vi "Finish.vi"   [LabVIEW 2012]
doc: "This VI is called just before exiting. It is expected to close I/O refnum, save collected data, etc."
uses:
  <vilib>/Rock Robotics/WPI/RobotDrive/WPI_RobotDriveGetSetRefNum.vi
  <vilib>/Rock Robotics/WPI/Joystick/WPI_JoystickGetSetRefNum.vi
types:
  T1 = typedef "WPI_SolenoidDevRef.ctl" = cluster{"DevStatus":errorcluster, "Solenoid Module":T2, "Forward Solenoid Channel":T3, "Reverse Solenoid Channel":T3}
  T2 = typedef "FPGA_TypedefSolenoidModule.ctl" = enum16{"Solenoid Module 1", "Solenoid Module 2"}
  T3 = typedef "WPI_SolenoidChannel.ctl" = enum8{"Solenoid 1", "Solenoid 2", "Solenoid 3", "Solenoid 4", "Solenoid 5", "Solenoid 6", "Solenoid 7", "Solenoid 8", "Invalid"}
  T4 = typedef "WPI_JoystickDevRef.ctl" = cluster{"Device":T5}
  T5 = typedef "WPI_JoystickDeviceEnum.ctl" = enum16{"USB 1", "USB 2", "USB 3", "USB 4", "Kinect 1", "Kinect 2"}
  T6 = typedef "WPI_RobotDriveDevRef.ctl" = cluster{"DevStatus":errorcluster, "Motors[]":T7[], "Square Inputs":bool, "Max Output":dbl, "Isochronous":bool}
  T7 = typedef "WPI_MotorControlDeviceRef.ctl" = cluster{"DeviceStatus":errorcluster, "Type":enum16{"PWM", "CAN"}, "PWM":cluster{"Digital Module":T8, "PWM Channel":T9, "DeadBand":T10}, "CAN":cluster{"Device Number":u8, "Control Mode":T11, "Semaphore":T12, "Max Vout":dbl}, "Invert":bool, "TransformRef":T13, "InvTransformRef":T13}
  T8 = typedef "FPGA_TypedefDigitalModule.ctl" = enum16{"Digital Module 1", "Digital Module 2"}
  T9 = typedef "FPGA_DIOPWMChannel.ctl" = enum8{"PWM 1", "PWM 2", "PWM 3", "PWM 4", "PWM 5", "PWM 6", "PWM 7", "PWM 8", "PWM 9", "PWM 10", "Invalid"}
  T10 = typedef "WPI_PWMDeadband.ctl" = cluster{"Name":string, "maxPositivePwm":i32, "minPositivePwm":i32, "centerPwm":i32, "maxNegativePwm":i32, "minNegativePwm":i32, "angularRange":u16}
  T11 = typedef "WPI_CANJaguar_ControlMode.ctl" = enum8{"Percent VBus", "Current", "Speed", "Position", "Voltage"}
  T12 = typedef "Semaphore RefNum" = refnum<k1>
  T13 = typedef "WPI_PWMTransform_ConPane.ctl" = refnum<vi>
  T14 = typedef "WPI_CameraDevRef.ctl" = cluster{"Camera Address":string, "CameraStatus":errorcluster, "Acquire Image Notifier":refnum<notifier>}
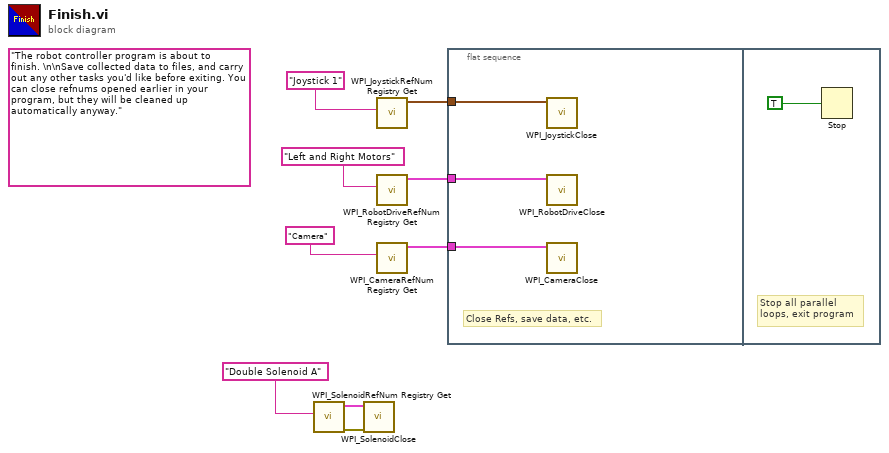
[diagram p0: block diagram]
diagram:
  (unwired) "The robot controller program is about to finish. \n\nSave collected data to files, and carry out any other tasks you'd like before exiting. You can close refnums opened earlier in your program, but they will be cleaned up automatically anyway."
  n1 = call <vilib>:"WPI_SolenoidRefNum Registry Get.vi"("refnum name"="Double Solenoid A") -> ("error out"=w2:errorcluster, "SolenoidDevRef"=w3:T1)  [unwired: 9 in]
  n2 = call <vilib>:"WPI_SolenoidClose.vi"("error in (no error)"=w2, "SolenoidDevRef"=w3) -> ()  [unwired: 9 in, 1 out]
  n3 = call <vilib>:"WPI_JoystickRefNum Registry Get.vi"("refnum name"="Joystick 1") -> ("JoystickDevRef"=w6:T4)  [unwired: 1 in, 9 out]
  n4 = call <vilib>:"WPI_RobotDriveRefNum Registry Get.vi"("refnum name"="Left and Right Motors") -> ("RobotDriveDevRef"=w7:T6)  [unwired: 1 in, 9 out]
  n5 = call <vilib>:"WPI_CameraRefNum Registry Get.vi"("refnum name"="Camera") -> ("CameraDevRef"=w5:T14)  [unwired: 1 in, 9 out]
  n6 = flat-sequence {
    tunnel: w7 -> [w12]
    tunnel: w6 -> [w11]
    tunnel: w5 -> [w10]
    frame #0 {
      # "Close Refs, save data, etc."
      n7 = call <vilib>:"WPI_JoystickClose.vi"("JoystickDevRef"=w11) -> ()  [unwired: 11 out]
      n8 = call <vilib>:"WPI_RobotDriveClose.vi"("RobotDriveDevRef"=w12) -> ()  [unwired: 1 in, 10 out]
      n9 = call <vilib>:"WPI_CameraClose.vi"("CameraDevRef"=w10) -> ()  [unwired: 1 in, 10 out]
    }
    frame #1 {
      # "Stop all parallel\nloops, exit program"
      n10 = Stop(stop? (T)=TRUE ("Quit")) -> ()
    }
  }
